vi "DBC Op.vi"(8 "error in (no error)":errorcluster, 9 "payload":u8[](array[numeric])=[140, 5, 0, 0, 0, 205, 218, 172, 202, 134, 212, 0, 0, 0, 0, 0, 20, 6, 0, 0, 0, 205, 214, 171, 199, 128, 12, 0, 0, 0, 0, 0, 107, 6, 0, 0, 0, 205, 86, 79, 7, 253, 54, 0, 0, 0, 0, 0, 0, 0, 0, 0, 0, 0, 0, 0, 0, 0, 0, 0, 0, 0, 0, 0] format="%.0x", 10 "ID":u32=1024 format="%.0x", 11 "Enum":enum16{"Init", "GetData", "Clear"}(ring)) -> (0 "error out":errorcluster, 2 "signal data":dbl[](array[numeric])=[1.0, -0.87, 0.0, 0.0, 0.27, 0.0, 0.0, 0.0, 0.0, -101.0, 14.200000000000001, 0.0, 27.32, -74.0, 0.0, 1.0, 0.25, 0.0, 0.0, 0.03, 0.0, 0.0, 0.0, 0.0, -101.0, 15.56, 0.0, 19.63, -82.0, 0.0, 0.0, 1.09, 0.0, 0.0, -0.12, 0.0, 0.0, 0.0, 0.0, -101.0, 16.43, 0.0, 18.71, -82.0, 0.0, 0.0, 0.0, 0.0, 0.0, 0.0, 0.0, 0.0, 0.0, 0.0, -255.0, 0.0, 0.0, 0.0, -255.0, 0.0] format="%.2f", 3 "signals":string[](array[string])=["LGU1_azAmb", "LGU1_azAngle", "LGU1_azAngleQly", "LGU1_elAmb", "LGU1_elAngle", "LGU1_elAngleQly", "LGU1_existProb", "LGU1_locPeerIdx", "LGU1_measStatus", "LGU1_noi", "LGU1_radDist", "LGU1_radVel", "LGU1_rcsEst", "LGU1_sigPwr", "LGU1_velQly", "LGU2_azAmb", "LGU2_azAngle", "LGU2_azAngleQly", "LGU2_elAmb", "LGU2_elAngle", "LGU2_elAngleQly", "LGU2_existProb", "LGU2_locPeerIdx", "LGU2_measStatus", "LGU2_noi", "LGU2_radDist", "LGU2_radVel", "LGU2_rcsEst", "LGU2_sigPwr", "LGU2_velQly", "LGU3_azAmb", "LGU3_azAngle", "LGU3_azAngleQly", "LGU3_elAmb", "LGU3_elAngle", "LGU3_elAngleQly", "LGU3_existProb", "LGU3_locPeerIdx", "LGU3_measStatus", "LGU3_noi", "LGU3_radDist", "LGU3_radVel", "LGU3_rcsEst", "LGU3_sigPwr", "LGU3_velQly", "LGU4_azAmb", "LGU4_azAngle", "LGU4_azAngleQly", "LGU4_elAmb", "LGU4_elAngle", "LGU4_elAngleQly", "LGU4_existProb", "LGU4_locPeerIdx", "LGU4_measStatus", "LGU4_noi", "LGU4_radDist", "LGU4_radVel", "LGU4_rcsEst", "LGU4_sigPwr", "LGU4_velQly"])   [LabVIEW 2024]
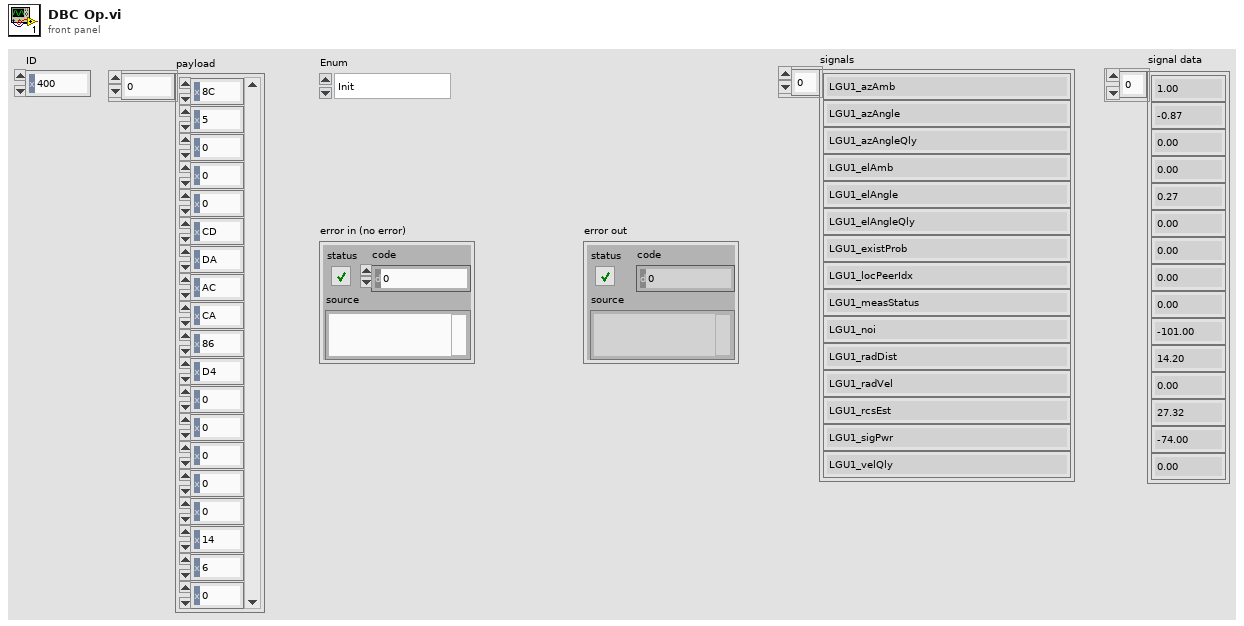
[diagram p1: front panel]
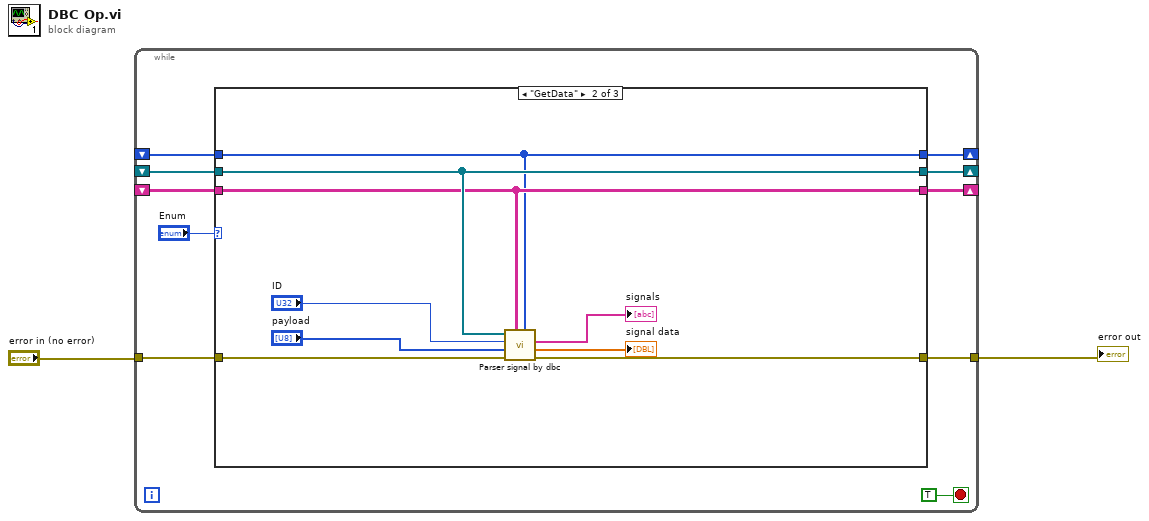
[diagram p0: block diagram]
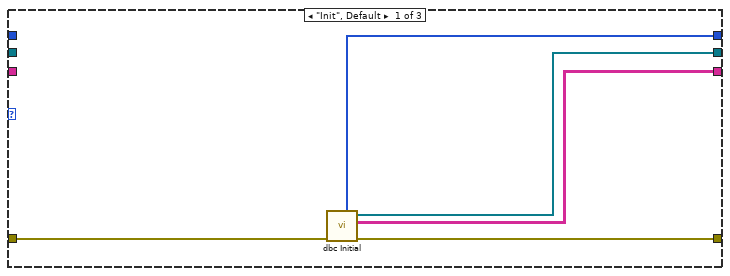
[diagram p2: hidden frame]
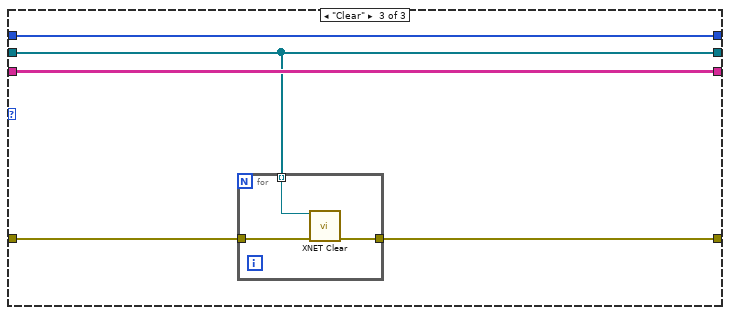
[diagram p3: hidden frame]
diagram:
  n1 = while {
    tunnel: [w12] -> w2
    tunnel: "error in (no error)" -> [w10]
    shift-right: [w8] -> _
    shift-left: _ -> [w5]
    shift-right: [w9] -> _
    shift-left: _ -> [w6]
    shift-right: [w4] -> _
    shift-left: _ -> [w3]
    stop <- TRUE stop-if-true
    n2 = case shown="\"GetData\"" "Enum" {
      tunnel: [w17 w25 w29] -> w12
      tunnel: w10 -> [w16 w26 w30]
      tunnel: [w15 w24 w28] -> w9
      tunnel: [w14 w23 w31] -> w8
      tunnel: w6 -> [_ w24 w28]
      tunnel: w5 -> [_ w23 w31]
      tunnel: [w13 w18 w27] -> w4
      tunnel: w3 -> [_ w18 w27]
      frame "Init", Default {
        n3 = call "dbc Initial.vi"("error in (no error)"=w16) -> ("error out"=w17:errorcluster, "NameShort"=w14:string[][], "Session Out"=w15:refnum<k21>[], "ID"=w13:u32[])  [unwired: 7 in]
      }
      frame "GetData" {
        n4 = call "Parser signal by dbc.vi"("ID array"=w18, "NameShort"=w23, "error in (no error)"=w26, "payload"="payload", "ID"="ID", "Session"=w24) -> ("error out"=w25:errorcluster, "signal data"=→"signal data":dbl[], "Names"=→"signals":string[])  [unwired: 3 in]
      }
      frame "Clear" {
        n5 = for {
          tunnel: w30 -> [w34]
          tunnel: [w33] -> w29
          tunnel: w28 -> [w32] mode=indexing
          n6 = call <vilib>:"XNET Clear.vi"("session in"=w32, "error in (no error)"=w34) -> ("error out"=w33:errorcluster)  [unwired: 13 in]
        }
      }
    }
  }
  "error out" <- w2
